vi "velosterlcmpaser.vi"() -> (2 "mdps torque":dbl)   [LabVIEW 2015]
uses:
  G_LCM.vi
  G_ALL.vi
panel:
  in  "x":dbl
  in  "y":dbl
  out "Waveform Chart":dynamicdata(graph)
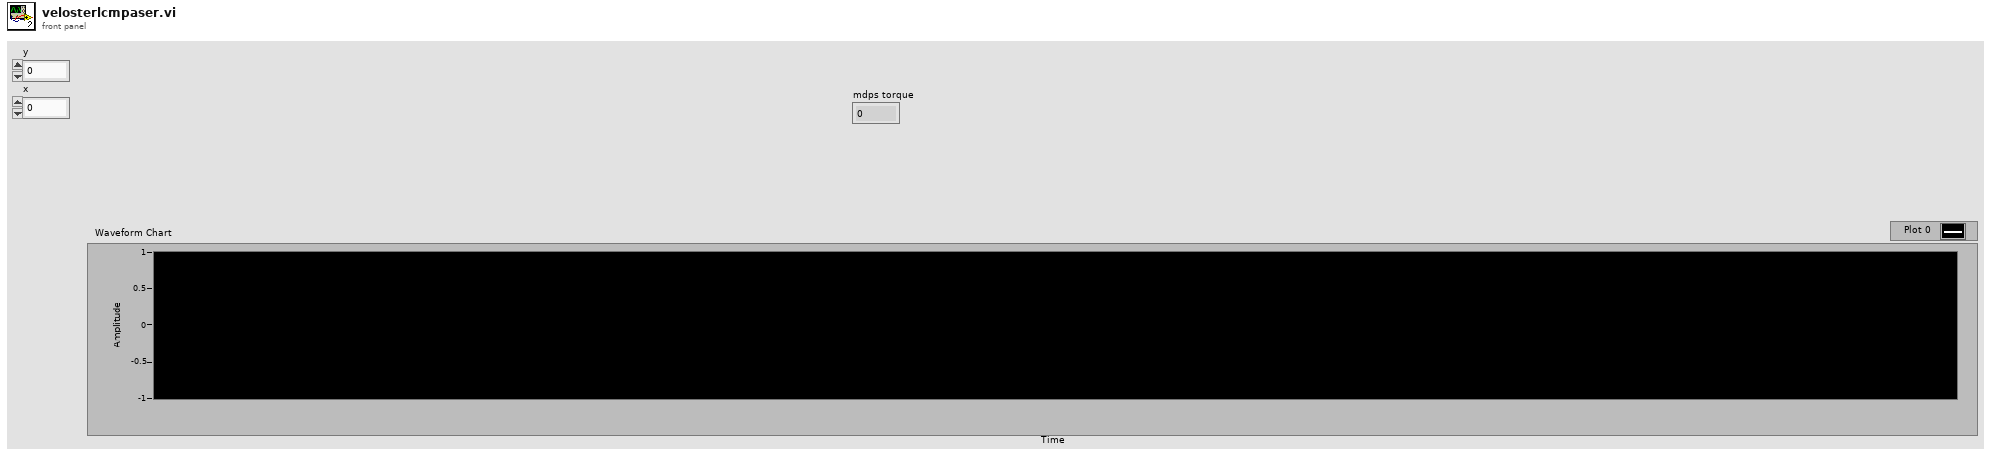
[diagram p1: front panel]
types:
  T1 = cluster{"hash":i64, "sys time":i64, "n":u32, "pathxy":dbl[]}
  T2 = cluster{"C_Wheel base":dbl, "ratio_steer":dbl, "Overall width":dbl, "af":dbl, "turn radius":dbl, "eval":dbl, "ap":dbl, "an":dbl, "Vmax":dbl, "mu":dbl, "Vlast":dbl}
  T3 = cluster{"hash":i64, "sys time":i64, "Auto":bool, "Run":bool, "Solenoid":bool, "T lim":bool, "brk_enc":u8, "B PWM":u16, "T PWM":u16, "ref_vel":dbl, "ref_bkr_enc":dbl, "ref_apv":dbl, "ref_steer":dbl}
  T4 = cluster{"hash":i64, "sys time":i64, "time":dbl, "yaw_rate":dbl, "mdps torque":dbl, "mdps str_ang":dbl, "VS_CAN":dbl, "lat_accel":dbl, "mcp":dbl, "accel pedal value":dbl, "tps":dbl, "odometer":dbl, "battery voltage":dbl, "WHL_SPD_RR":dbl, "WHL_SPD_RL":dbl, "WHL_SPD_FR":dbl, "WHL_SPD_FL":dbl}
  T5 = cluster{"hash":i64, "sys time":i64, "time":dbl, "x":dbl, "y":dbl, "h":dbl, "numSV":i32, "postype":i32, "lag":i32, "hordev":dbl, "lat":dbl, "lon":dbl, "hgt":dbl, "map_idx":i32}
  T6 = cluster{"hash":i64, "sys time":i64, "dt":dbl, "x":dbl, "y":dbl, "speed":dbl, "heading":dbl, "yaw_rate":dbl}
  T7 = cluster{"hash":dbl, "sys time":dbl, "time":dbl, "x":dbl, "y":dbl, "h":dbl, "numSV":dbl, "postype":dbl, "lag":dbl, "hordev":dbl, "lat":dbl, "lon":dbl, "hgt":dbl, "map_idx":dbl}
  T8 = cluster{"Steer_input":dbl, "Steer_output":dbl, "VS_des":dbl, "VS_can":dbl, "heading":dbl, "auto":bool, "run":bool, "x":dbl, "y":dbl}
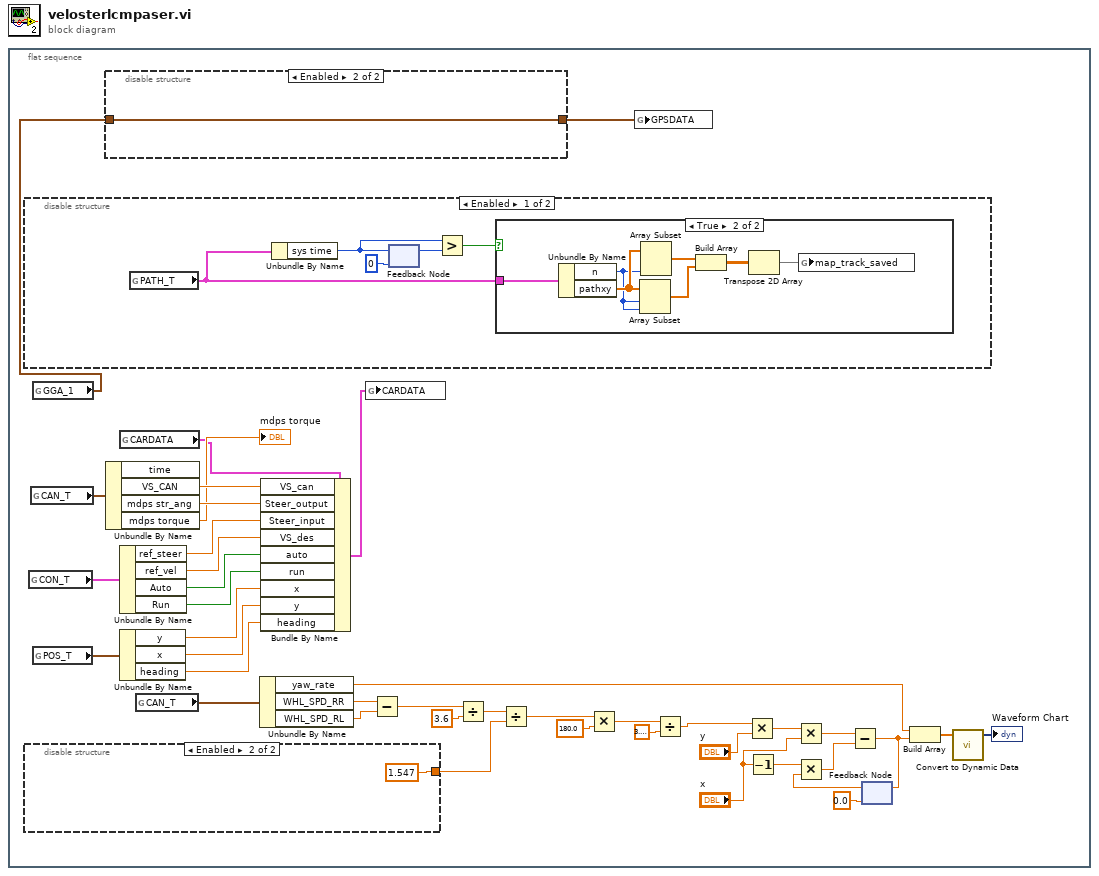
[diagram p0: block diagram]
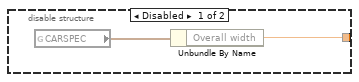
[diagram p2: hidden frame]
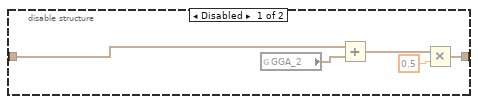
[diagram p5: hidden frame]
diagram:
  n1 = flat-sequence {
    frame #0 {
      n2 = disable-structure shown="Enabled" {
        frame Enabled {
          n3 = global read "G_LCM.vi" "PATH_T"() -> (w45:T1)
          n4 = Unbundle By Name(w45) -> ("sys time"=w48:i64)
          n5 = feedback #1(i64 0 ("sys time")) -> (w47:i64)
          n6 = feedback-in #1(w48) -> ()
          n7 = Greater?(x=w48, y=w47) -> (0:w49:bool)
          n8 = case shown="True" w49 {
            tunnel: w45 -> [_ w50]
            frame False {
            }
            frame True {
              n9 = Unbundle By Name(w50) -> ("n"=w55:u32, "pathxy"=w56:dbl[])
              n10 = Array Subset(array=w56, index=w55, length=w55) -> (w53:dbl[])
              n11 = Array Subset(array=w56, length=w55) -> (w54:dbl[])  [unwired: 1 in]
              n12 = Build Array(w54, w53) -> (w52:dbl[][])
              n13 = Transpose 2D Array(2D array=w52) -> (transposed array=w51:dbl[][])
              n14 = global write "G_ALL.vi" "map_track_saved"(w51) -> ()
            }
          }
        }
        frame Disabled {
        }
      }
      n15 = disable-structure shown="Enabled" {
        disable-tunnel: [w42 1.547 ("Overall width")] -> w19
        frame Disabled {
          n16 = global read "G_ALL.vi" "CARSPEC"() -> (w43:T2)
          n17 = Unbundle By Name(w43) -> ("Overall width"=w42:dbl)
        }
        frame Enabled {
        }
      }
      n18 = global read "G_LCM.vi" "CON_T"() -> (w40:T3)
      n19 = global read "G_LCM.vi" "CAN_T"() -> (w41:T4)
      n20 = global read "G_LCM.vi" "GGA_1"() -> (w29:T5)
      n21 = global read "G_LCM.vi" "POS_T"() -> (w1:T6)
      n22 = disable-structure shown="Enabled" {
        disable-tunnel: w29 -> [w61 w62]
        disable-tunnel: [w57 w62] -> w26
        frame Disabled {
          n23 = global read "G_LCM.vi" "GGA_2"() -> (w60:T5)
          n24 = Add(x=w61, y=w60) -> (x+y=w59:T5)
          n25 = Multiply(x=w59, y=0.5) -> (x*y=w57:T7)
        }
        frame Enabled {
        }
      }
      n26 = Unbundle By Name(w41) -> ("VS_CAN"=w32:dbl, "mdps str_ang"=w37:dbl, "mdps torque"=→"mdps torque":dbl)  [unwired: 1 out]
      n27 = global read "G_ALL.vi" "CARDATA"() -> (w27:T8)
      n28 = Unbundle By Name(w40) -> ("ref_steer"=w33:dbl, "ref_vel"=w34:dbl, "Auto"=w35:bool, "Run"=w36:bool)
      n29 = Unbundle By Name(w1) -> ("y"=w39:dbl, "x"=w38:dbl, "heading"=w31:dbl)
      n30 = global read "G_LCM.vi" "CAN_T"() -> (w25:T4)
      n31 = Unbundle By Name(w25) -> ("yaw_rate"=w18:dbl, "WHL_SPD_RR"=w24:dbl, "WHL_SPD_RL"=w23:dbl)
      n32 = Bundle By Name(cluster=w27, "VS_can"=w32, "Steer_output"=w37, "Steer_input"=w33, "VS_des"=w34, "auto"=w35, "run"=w36, "x"=w39, "y"=w38, "heading"=w31) -> (w28:T8)
      n33 = global write "G_ALL.vi" "CARDATA"(w28) -> ()
      n34 = Subtract(x=w24, y=w23) -> (x-y=w22:dbl)
      n35 = Divide(x=w22, y=3.6) -> (x/y=w20:dbl)
      n36 = Divide(x=w20, y=w19) -> (x/y=w15:dbl)
      n37 = Multiply(x=w15, y=180.0) -> (x*y=w13:dbl)
      n38 = global write "G_ALL.vi" "GPSDATA"(w26) -> ()
      n39 = Divide(x=w13, y=3.141592653589793) -> (x/y=w11:dbl)
      n40 = Multiply(x=w11, y="y") -> (x*y=w9:dbl)
      n41 = Decrement(x="x") -> (x-1=w6:dbl)
      n42 = Multiply(x=w9, y="x") -> (x*y=w8:dbl)
      n43 = feedback #2(0.0) -> (w5:dbl)
      n44 = Multiply(x=w6, y=w5) -> (x*y=w4:dbl)
      n45 = Subtract(x=w8, y=w4) -> (x-y=w2:dbl)
      n46 = feedback-in #2(w2) -> ()
      n47 = Build Array(w18, w2) -> (w17:dbl[])
      n48 = call "Convert to Dynamic Data"("Array"=w17) -> ("Dynamic Data Type"=→"Waveform Chart":dynamicdata)  [unwired: 3 in]
    }
  }
